vi "OpenConnectionToIrDAServer.vi"() -> (0 "error out":errorcluster, 2 "IrDA Refnum":refnum<k19>)   [LabVIEW 2010]
doc: "And the description is..."
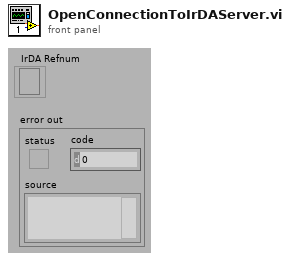
[diagram p1: front panel]
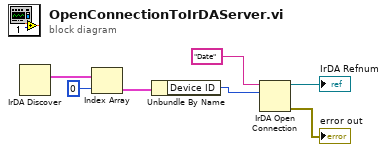
[diagram p0: block diagram]
diagram:
  n1 = IrDA Discover() -> (2:w7:cluster{"Device ID":u32, "Device Name":string}[])  [unwired: 1 in, 2 out]
  n2 = Index Array(array=w7, index=0) -> (element=w5:cluster{"Device ID":u32, "Device Name":string})
  n3 = Unbundle By Name(w5) -> ("Device ID"=w4:u32)
  n4 = IrDA Open Connection(10:w4, 11:"Date" ("service name")) -> (0:→"error out":errorcluster, 3:→"IrDA Refnum":refnum<k19>)  [unwired: 1 in, 1 out]
